vi "双容水槽1111.vi"() -> ()   [LabVIEW 2013]
panel:
  out "阀 3":bool
  in  "最小水位 2":u8=25
  in  "最小水位":u8=25
  in  "执行":bool
  out "水管 4":bool
  out "水管2":bool
  out "阀 2":bool
  out "阀1":bool
  out "水管5":T1
  in  "最大水位2":u8=85 min=25 max=100
  in  "最大水位":u8=80 min=25 max=100
  out "水管3":T1
  out "水管1":T1
  out "水箱 2":dbl(slide) scale=0.0..100.0
  out "水箱1":dbl(slide) scale=0.0..100.0
  # "双容水槽仿真系统"
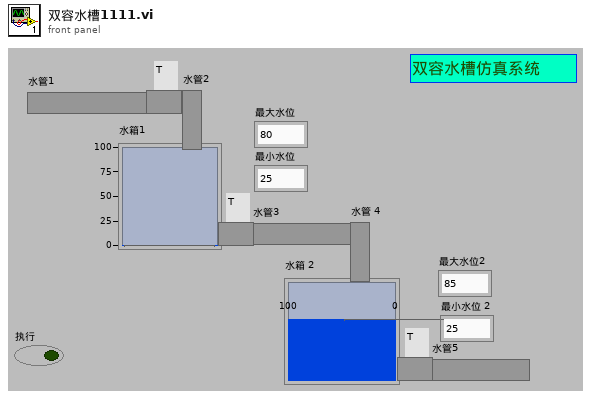
[diagram p1: front panel]
types:
  T1 = typedef "水管1.ctl" = bool
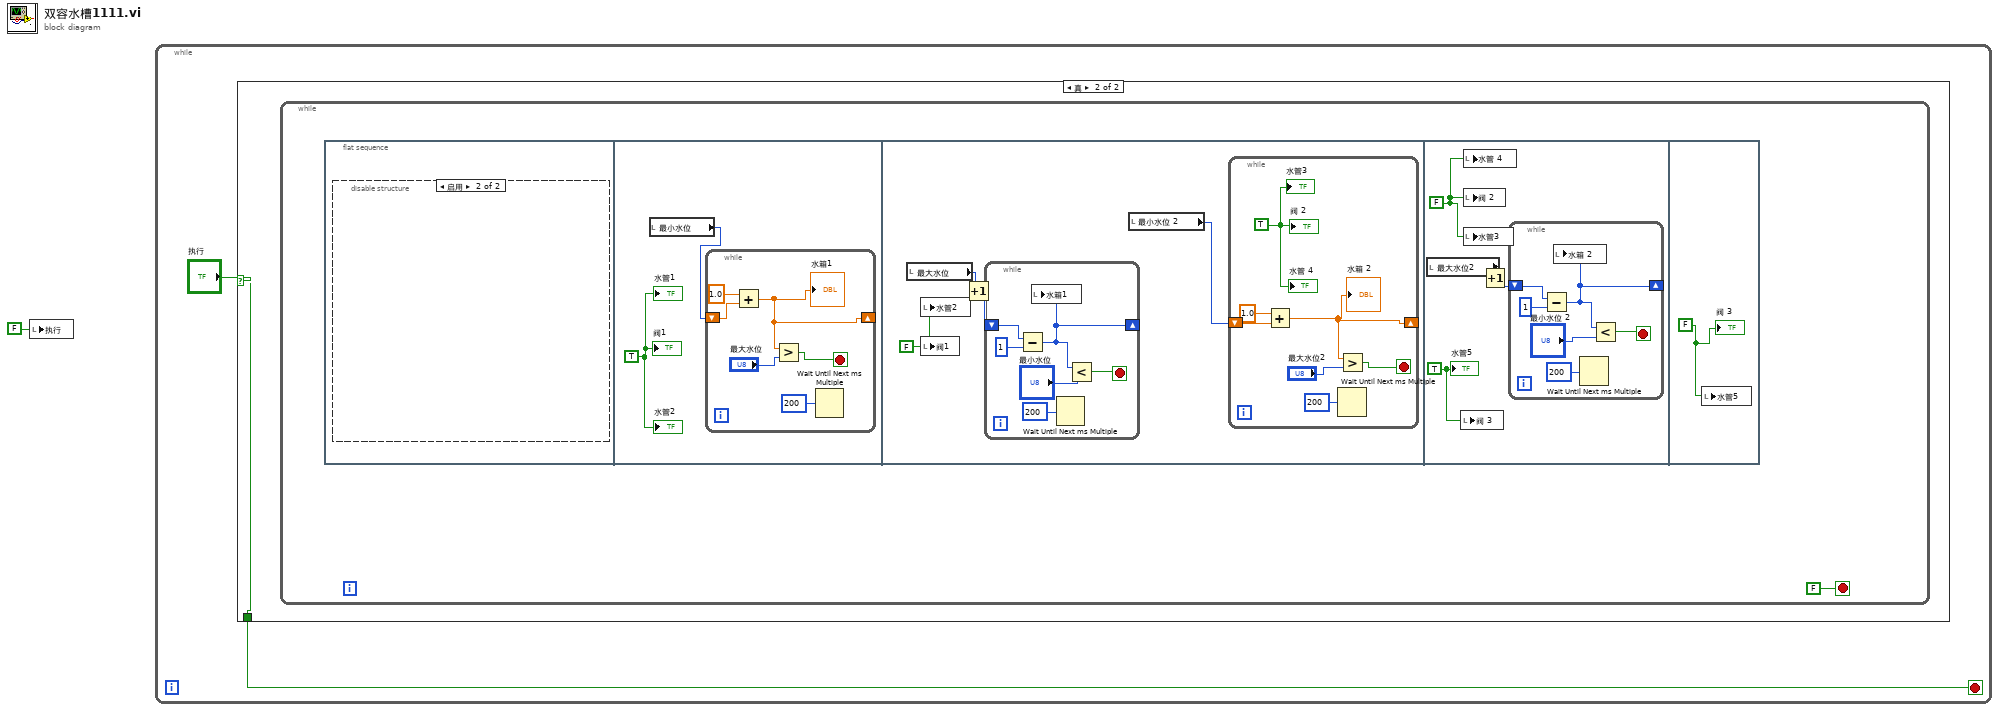
[diagram p0: block diagram]
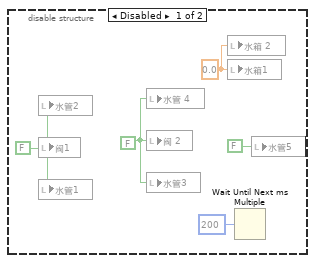
[diagram p3: hidden frame]
diagram:
  n1 = local write "执行"(FALSE ("执行")) -> ()
  n2 = while {
    stop <- w2 stop-if-true
    n3 = case shown="真" "执行" {
      selector: "执行" -> [_ w4]
      tunnel: [_ w4] -> w2
      frame False {
      }
      frame True {
        n4 = while {
          stop <- FALSE stop-if-true
          n5 = flat-sequence {
            frame #0 {
              n6 = disable-structure shown="启用" {
                frame Disabled {
                  w7 = 0.0 ("水箱1")
                  w9 = FALSE
                  w10 = FALSE
                  n7 = local write "水管2"(w9) -> ()
                  n8 = local write "阀1"(w9) -> ()
                  n9 = local write "水管1"(w9) -> ()
                  n10 = local write "水管 4"(w10) -> ()
                  n11 = local write "阀 2"(w10) -> ()
                  n12 = local write "水管3"(w10) -> ()
                  n13 = local write "水箱 2"(w7) -> ()
                  n14 = local write "水箱1"(w7) -> ()
                  n15 = Wait Until Next ms Multiple(millisecond multiple=u32 200 ("毫秒倍数")) -> ()  [unwired: 1 out]
                  n16 = local write "水管5"(T1 FALSE ("水管5")) -> ()
                }
                frame Enabled {
                }
              }
            }
            frame #1 {
              w12 = TRUE
              n17 = local read "最小水位"() -> (w11:u8)
              n18 = while {
                shift-right: [w15] -> _
                shift-left: w11 -> [w18]
                stop <- w14 stop-if-true
                n19 = Add(x=1.0, y=w18) -> (x+y=w15:dbl)
                "水箱1" <- w15
                n20 = Greater?(x=w15, y="最大水位") -> (0:w14:bool)
                n21 = Wait Until Next ms Multiple(millisecond multiple=u32 200 ("毫秒倍数")) -> ()  [unwired: 1 out]
              }
              "水管1" <- w12
              "阀1" <- w12
              "水管2" <- w12
            }
            frame #2 {
              w20 = FALSE
              n22 = local read "最大水位"() -> (w21:u8)
              n23 = local write "水管2"(w20) -> ()
              n24 = local write "阀1"(w20) -> ()
              n25 = Increment(x=w21) -> (x+1=w22:u8)
              n26 = while {
                shift-right: [w33] -> _
                shift-left: w22 -> [w35]
                stop <- w32 stop-if-true
                n27 = Subtract(x=w35, y=u8 1) -> (x-y=w33:u8)
                n28 = local write "水箱1"(w33) -> ()
                n29 = Wait Until Next ms Multiple(millisecond multiple=u32 200 ("毫秒倍数")) -> ()  [unwired: 1 out]
                n30 = Less?(x=w33, y="最小水位") -> (x < y?=w32:bool)
              }
              n31 = local read "最小水位 2"() -> (w19:u8)
              n32 = while {
                shift-right: [w24] -> _
                shift-left: w19 -> [w28]
                stop <- w25 stop-if-true
                w23 = TRUE
                n33 = Add(x=1.0, y=w28) -> (x+y=w24:dbl)
                "水箱 2" <- w24
                n34 = Greater?(x=w24, y="最大水位2") -> (0:w25:bool)
                n35 = Wait Until Next ms Multiple(millisecond multiple=u32 200 ("毫秒倍数")) -> ()  [unwired: 1 out]
                "水管3" <- w23
                "阀 2" <- w23
                "水管 4" <- w23
              }
            }
            frame #3 {
              w37 = FALSE ("阀 2")
              w36 = T1 TRUE ("水管5")
              n36 = local read "最大水位2"() -> (w38:u8)
              n37 = local write "阀 3"(w36) -> ()
              n38 = local write "水管 4"(w37) -> ()
              n39 = local write "阀 2"(w37) -> ()
              n40 = local write "水管3"(w37) -> ()
              n41 = Increment(x=w38) -> (x+1=w39:u8)
              n42 = while {
                shift-right: [w43] -> _
                shift-left: w39 -> [w45]
                stop <- w42 stop-if-true
                n43 = Subtract(x=w45, y=u8 1) -> (x-y=w43:u8)
                n44 = local write "水箱 2"(w43) -> ()
                n45 = Wait Until Next ms Multiple(millisecond multiple=u32 200 ("毫秒倍数")) -> ()  [unwired: 1 out]
                n46 = Less?(x=w43, y="最小水位 2") -> (x < y?=w42:bool)
              }
              "水管5" <- w36
            }
            frame #4 {
              w46 = FALSE ("阀 2")
              n47 = local write "水管5"(w46) -> ()
              "阀 3" <- w46
            }
          }
        }
      }
    }
  }
